vi "Write Port simulated.vi"(8 "error in (no error)":errorcluster, 9 "Port 2":dbl, 10 "Binary Number":T1, 11 "Simulated Device in":refnum<class "Simulated Device.lvclass">) -> (0 "error out":errorcluster, 1 "Response":string, 3 "Simulated Device out":refnum<class "Simulated Device.lvclass">)   [LabVIEW 2020, in "Simulated Device.lvclass"]
uses:
  Simulated Device.lvclass
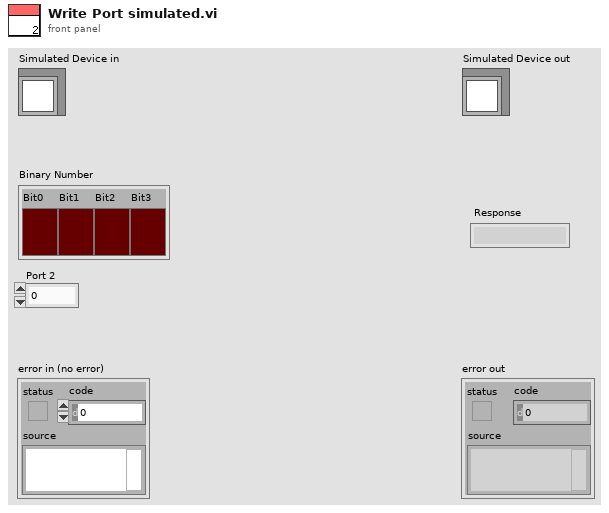
[diagram p1: front panel]
types:
  T1 = cluster{"Bit0":bool, "Bit1":bool, "Bit2":bool, "Bit3":bool}
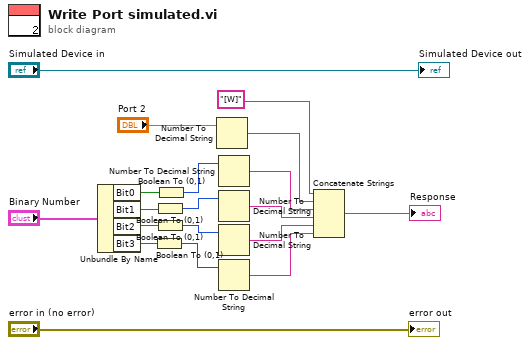
[diagram p0: block diagram]
diagram:
  n1 = Unbundle By Name("Binary Number") -> ("Bit0"=w17:bool, "Bit1"=w16:bool, "Bit2"=w15:bool, "Bit3"=w14:bool)
  n2 = Boolean To (0,1)(Boolean=w14) -> (0, 1=w12:i16)
  n3 = Boolean To (0,1)(Boolean=w16) -> (0, 1=w10:i16)
  n4 = Boolean To (0,1)(Boolean=w15) -> (0, 1=w11:i16)
  n5 = Boolean To (0,1)(Boolean=w17) -> (0, 1=w13:i16)
  n6 = Number To Decimal String(number="Port 2") -> (decimal integer string=w2:string)  [unwired: 1 in]
  n7 = Number To Decimal String(number=w13) -> (decimal integer string=w9:string)  [unwired: 1 in]
  n8 = Number To Decimal String(number=w10) -> (decimal integer string=w8:string)  [unwired: 1 in]
  n9 = Number To Decimal String(number=w11) -> (decimal integer string=w7:string)  [unwired: 1 in]
  n10 = Number To Decimal String(number=w12) -> (decimal integer string=w6:string)  [unwired: 1 in]
  n11 = Concatenate Strings("[W]" ("string"), w2, w9, w8, w7, w6) -> (→"Response":string)
  "error out" <- "error in (no error)"
  "Simulated Device out" <- "Simulated Device in"
